vi "Do.vi"(8 "error in (no error)":errorcluster, 10 "Actor in":refnum<class "Actor.lvclass">, 11 "Change Mixer Speed Msg":refnum<class "Change Mixer Speed Msg.lvclass">) -> (0 "error out":errorcluster, 2 "Actor out":refnum<class "Actor.lvclass">)   [LabVIEW 2018, in "Feeder Actor.lvlib" / "Change Mixer Speed Msg.lvclass"]
doc: "This VI delivers the message to the actor by calling the appropriate method(s) on the actor."
uses:
  Change Mixer Speed Msg.lvclass
  <vilib>/ActorFramework/Actor/Actor.lvclass
  Mixer/Mixer.lvclass
  Change Mixer Speed Msg.lvclass/Change Mixer Speed Msg.ctl
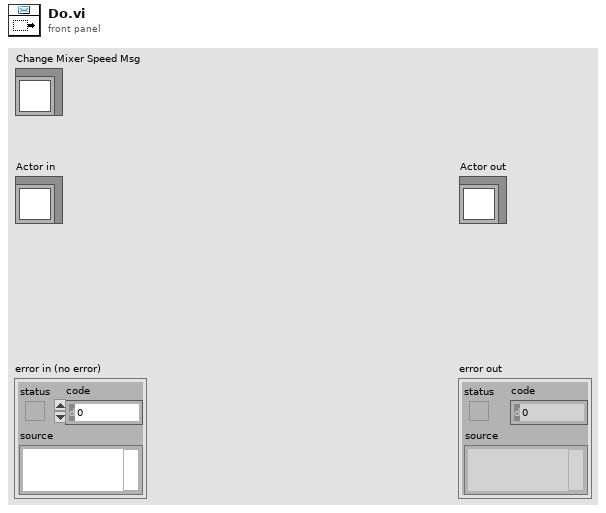
[diagram p1: front panel]
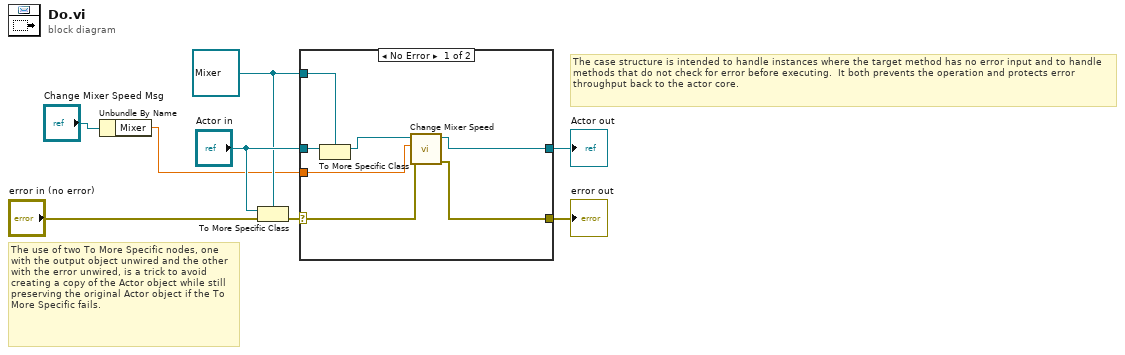
[diagram p0: block diagram]
diagram:
  w3 = refnum<class "Mixer.lvclass"> refnum ("Actor in")
  # "The use of two To More Specific nodes, one with the output object unwired and the other with the error unwired, is a trick to avoid creating a copy of the Actor object while still preserving the original Actor object if the To More Specific fails."
  # "The case structure is intended to handle instances where the target method has no error input and to handle methods that do not check for error before executing.  It both prevents the operation and protects error throughput back to the actor core."
  n1 = Unbundle By Name("Change Mixer Speed Msg") -> ("Mixer"=w1:dbl)
  n2 = To More Specific Class(target class=w3, reference="Actor in", error in="error in (no error)") -> (error out=w7:errorcluster)  [unwired: 1 out]
  n3 = case shown="No Error" w7 {
    selector: w7 -> [w11 w17]
    tunnel: [w10 w17] -> w6
    tunnel: [w9 w16] -> w5
    tunnel: "Actor in" -> [w15 w16]
    tunnel: w3 -> [w14 _]
    tunnel: w1 -> [w12 _]
    frame No Error {
      n4 = To More Specific Class(target class=w14, reference=w15) -> (specific class reference=w13:refnum<class "Mixer.lvclass">)  [unwired: 1 in, 1 out]
      n5 = call "Change Mixer Speed.vi"("error in (no error)"=w11, "Mixer"=w12, "Feeder Actor.lvlib:Mixer.lvclass"=w13) -> ("error out"=w10:errorcluster, "Actor out"=w9:refnum<class "Actor.lvclass">)  [unwired: 7 in]
    }
    frame Error {
      # "If type check fails, pass the original object out again."
    }
  }
  "error out" <- w6
  "Actor out" <- w5
